vi "例6-16.vi"() -> ()   [LabVIEW 2019]
uses:
  <vilib>/Analysis/3filter.llb/Filter Passband Type.ctl
  <vilib>/Analysis/3filter.llb/Butterworth Filter (DBL).vi
  <vilib>/Analysis/NI_AALBase.lvlib
panel:
  in  "停止":bool
  in  "阶数":dbl(slide)=5.1020408163265305 scale=0.0..10.0
  in  "截止频率":dbl(slide)=24.081632653061224 scale=0.0..40.0
  in  "采样点数":dbl=1000.0
  in  "采样频率":dbl=1000.0
  in  "正弦信号频率":dbl=5.0
  out "滤波后波形":cluster{i32, dbl, "Filtered X":dbl[]}(graph)
  out "滤波前波形":cluster{i32, dbl, dbl[]}(graph)
  # "信号参数设置"
  # "滤波器参数设置"
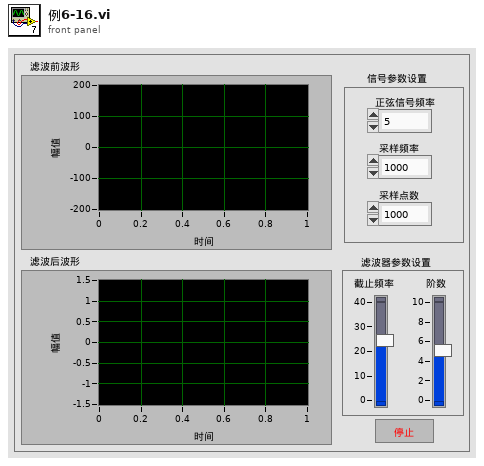
[diagram p1: front panel]
types:
  T1 = typedef "NI_AALBase.lvlib/Filter Passband Type.ctl" = enum32{"Lowpass", "Highpass", "Bandpass", "Bandstop"}
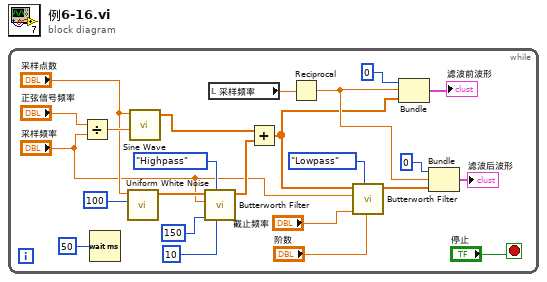
[diagram p0: block diagram]
diagram:
  n1 = while {
    stop <- "停止" stop-if-true
    n2 = Divide(x="正弦信号频率", y="采样频率") -> (x/y=w23:dbl)
    n3 = Wait (ms)(milliseconds to wait=50) -> ()  [unwired: 1 out]
    n4 = call <vilib>:"Uniform White Noise.vi"("amplitude"=100, "samples"="采样点数") -> ("uniform white noise"=w19:dbl[])  [unwired: 8 in, 1 out]
    n5 = call <vilib>:"Sine Wave.vi"("samples"="采样点数", "frequency"=w23) -> ("sine wave"=w20:dbl[])  [unwired: 3 in, 2 out]
    n6 = call-poly <vilib>:"Butterworth Filter.vi"("order"=10, "filter type"=Filter_Passband_Type."Highpass", "low cutoff freq: fl"=150, "sampling freq: fs"="采样频率", "X"=w19) -> ("Filtered X"=w15:dbl[])  [unwired: 3 in, 1 out]
    n7 = local read "采样频率"() -> (w8:dbl)
    n8 = Add(x=w20, y=w15) -> (x+y=w5:dbl[])
    n9 = Reciprocal(x=w8) -> (1/x=w7:dbl)
    n10 = call-poly <vilib>:"Butterworth Filter.vi"("order"="阶数", "filter type"=Filter_Passband_Type."Lowpass", "low cutoff freq: fl"="截止频率", "sampling freq: fs"="采样频率", "X"=w5) -> ("Filtered X"=w9:dbl[])  [unwired: 3 in, 1 out]
    n11 = Bundle(0, w7, w5) -> (→"滤波前波形":cluster{i32, dbl, dbl[]})  [unwired: 1 in]
    n12 = Bundle(0, w7, "Filtered X"=w9) -> (→"滤波后波形":cluster{i32, dbl, "Filtered X":dbl[]})  [unwired: 1 in]
  }
